vi "Firmware.vi"() -> ()   [LabVIEW 2017]
uses:
  <vilib>/Platform/TimedLoop/XDataNode/timing_clust.ctl
  <vilib>/Platform/TimedLoop/XDataNode/nitl_modes.ctl
  <vilib>/Platform/TimedLoop/XDataNode/wakeup.ctl
  <instrlib>/_niInstr/Instruction Framework/v1/FPGA/Helper Classes/Single Address Space Collection/Single Address Space Collection.lvclass
  C:/Program Files (x86)/National Instruments/LabVIEW 2017/instr.lib/_niInstr/Instruction Framework/v1/FPGA/Interfaces/Address Space Collection/Address Space Collection.lvclass
  <instrlib>/_niInstr/FIFO Register Bus/v1/FPGA/niInstr FIFO Register Bus v1 FPGA.lvclass
  C:/Program Files (x86)/National Instruments/LabVIEW 2017/instr.lib/_niInstr/Instruction Framework/v1/FPGA/Interfaces/Instruction Producer/Instruction Producer.lvclass
  <vilib>/rvi/Emulation/niFpgaGetClockAttributes.vi
  <vilib>/rvi/Emulation/niFpgaSctlEmulationGetInTimedLoop.vi
  <vilib>/rvi/Emulation/niFpgaEmulationReportErrorSimple.vi
  <vilib>/rvi/Emulation/niFpgaProcessEmulError.vi
  <vilib>/rvi/Emulation/niFpgaCriticalErrorInLSC.vi
  <vilib>/rvi/eio/common/nirviEmuTemplateMethod_errors.vi
  <vilib>/eio/EIONode/EIONode.xnode
  <vilib>/Platform/TimedLoop/XDataNode/XDataNode.xnode
  <instrlib>/_niInstr/Instruction Framework/v1/FPGA/Top Level Bus/Register Configuration/Register Configuration.lvclass
  <vilib>/Platform/TimedLoop/XDataNode/XDNodeRunTimeDep.lvlib
  <vilib>/NI/PowerElectronicsControl/ScaleAndLimit/Core/ScaleAndLimit.lvlib
  <vilib>/NI/PowerElectronicsControl/ScaleAndLimit/Core/AddressSpace.lvclass
  <vilib>/NI/PowerElectronicsControl/WaveformAcq/FPGA/WaveformAddressSpace.lvclass
panel:
  in  "ManualTrigger":bool
  out "TriggerTimestamp":i32
  out "FaultBuffer":u64 format="%.0x"
  out "relativeTimestamp":i32
  in  "fifo reg bus ctrl 0":u32
  out "fifo reg bus status 0":u32
  out "fifo reg bus data 0":u64
  out "SimultaneousAILoopRate":u32
  out "LimitsFlag":bool
  out "Simultaneous_AI":sgl[](array[numeric])
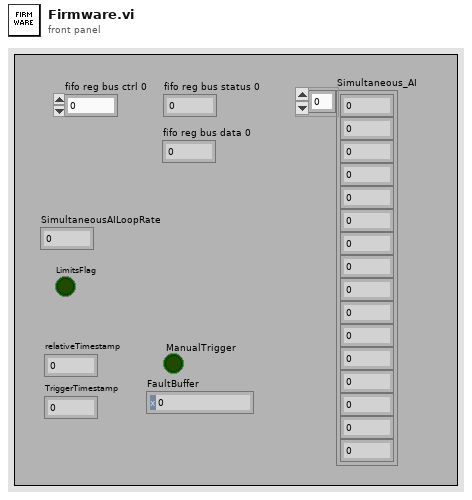
[diagram p1: front panel]
types:
  T1 = typedef "XDNodeRunTimeDep.lvlib/timing_clust.ctl" = cluster{"Expected End [f-1]":u64, "Actual End [f-1]":u64, "Finished Late? [f-1]":bool, "Expected End [i-1]":u64, "Actual End [i-1]":u64, "Finished Late? [i-1]":bool, "Expected Start [i]":u64, "Actual Start [i]":u64, "Expected Start [f]":u64, "Actual Start [f]":u64, "Source Name":string, "Structure Name":string, "Period":i64, "Deadline":i64, "Offset":i64, "Start":i64, "Priority":i32, "Timeout":i32, "Mode":T2, "Wakeup Reason":T3, "Error":errorcluster, "Source Type":string, "Secondary Source Type":string, "Global End Time":u64, "Global Start Time":u64, "Frame Duration":u64, "Iteration Duration":u64, "Assigned CPU":i32, "I/O Scan Engine Mode":u32}
  T2 = typedef "XDNodeRunTimeDep.lvlib/nitl_modes.ctl" = enum32{"No Change", "Process missed periods, maintain original phase", "Discard missed periods, maintain original phase", "Process missed periods, ignore original phase", "Discard missed periods, ignore original phase"}
  T3 = typedef "XDNodeRunTimeDep.lvlib/wakeup.ctl" = enum32{"Normal", "Aborted", "Asynchronous wakeup", "Timing source error", "Timed loop error", "Timeout"}
  T4 = typedef "ScaleAndLimit.lvlib/LimitsRegisters.ctl" = cluster{"HighLimits":refnum<k21>, "LowLimits":refnum<k21>, "ClearLimits":refnum<k21>, "LimitsFlag":refnum<k21>}
  T5 = typedef "ScaleAndLimit.lvlib/ConfigRegisters.ctl" = cluster{"LimitsEnabled":refnum<k21>, "UnscaledHighLimit":refnum<k21>, "UnscaledLowLimit":refnum<k21>, "B":refnum<k21>, "M":refnum<k21>}
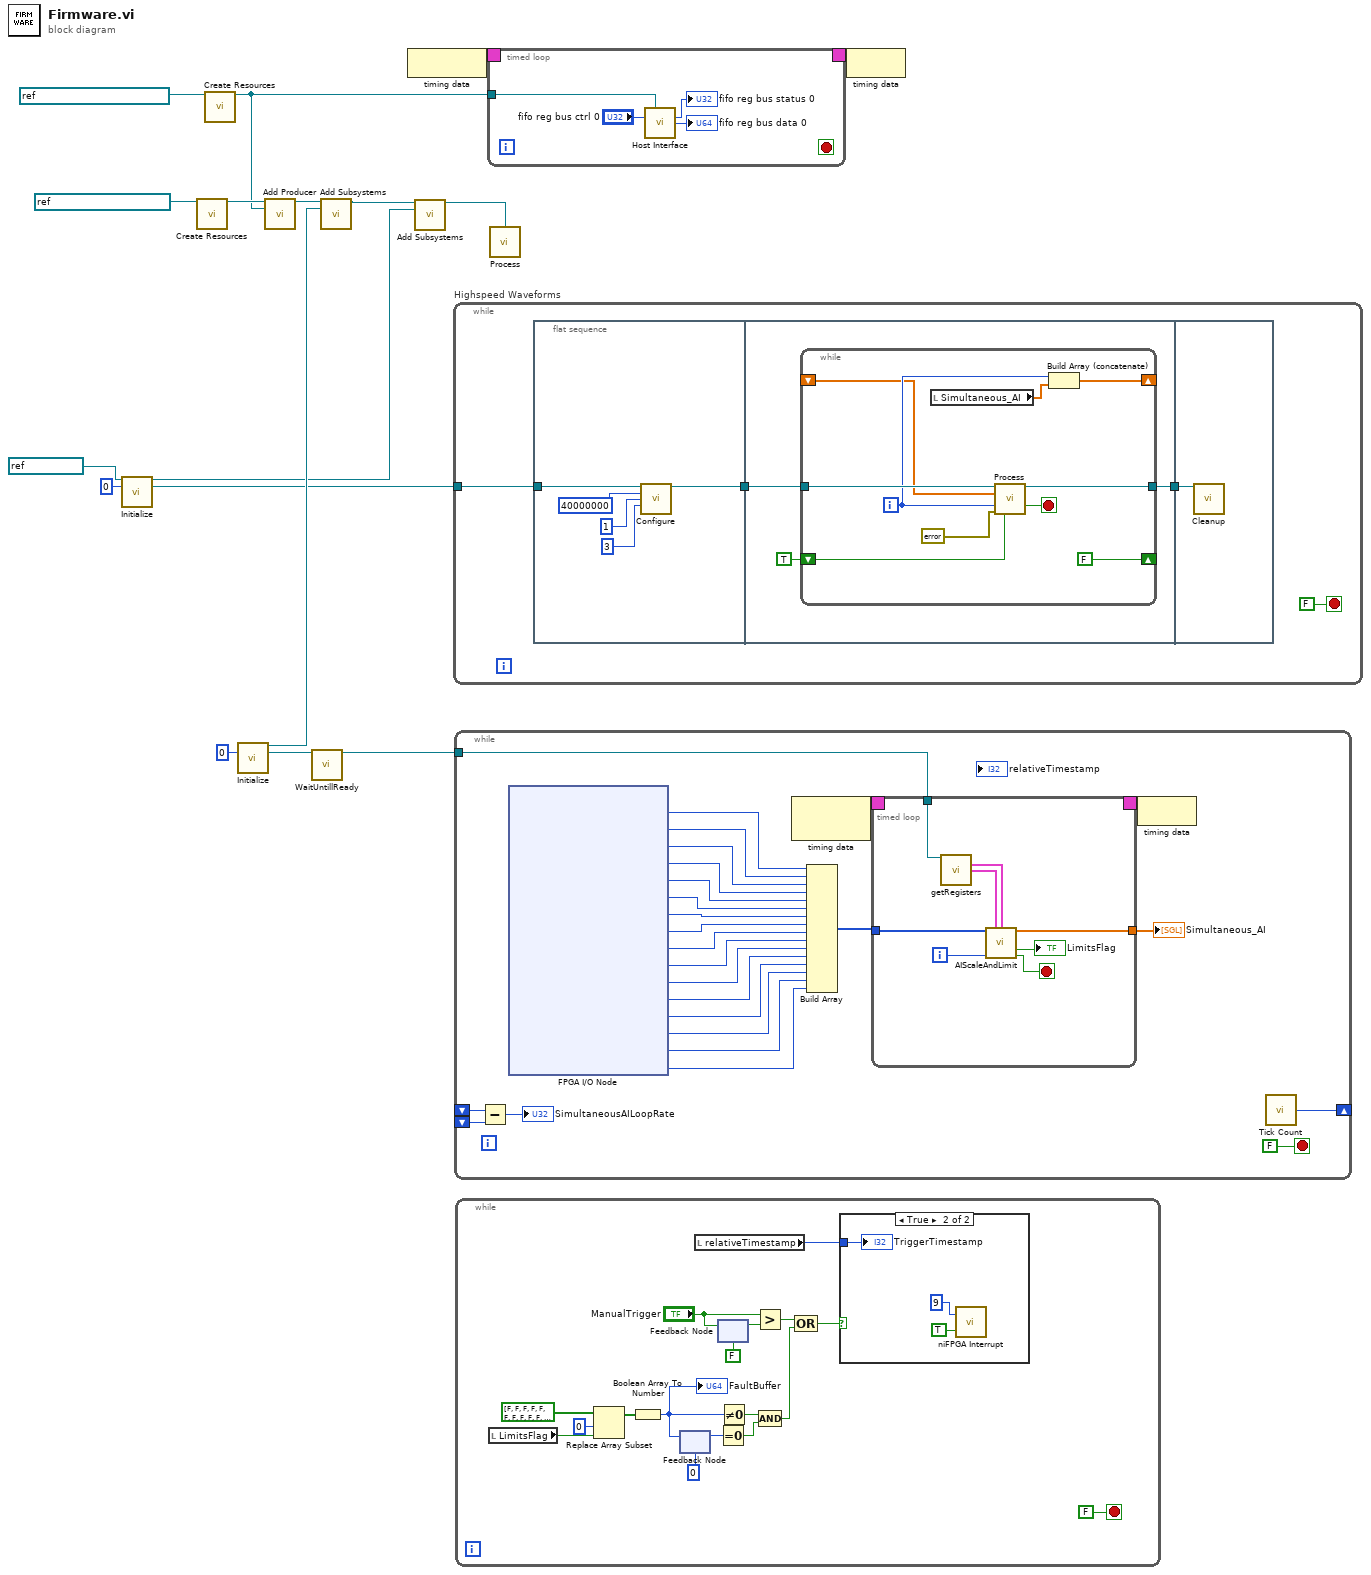
[diagram p0: block diagram]
diagram:
  n1 = call <vilib>:"Initialize.vi"("DMA FIFO"=refnum<k21> "DataSGL0" ("FIFO Out"), "instance"=u8 0) -> ("subsystem"=w3:refnum<class "Single Address Space Collection.lvclass">, "AddressSpace"=w6:refnum<class "WaveformAddressSpace.lvclass">)  [unwired: 12 in]
  n2 = call <instrlib>:"Create Resources.vi"("register clock"=refnum<k21> "40 MHz Onboard Clock") -> ("register configuration"=w15:refnum<class "Register Configuration.lvclass">)  [unwired: 14 in]
  n3 = call <instrlib>:"Create Resources.vi"("instruction fifo"=refnum<k21> "reg.host instruction fifo 0") -> ("fifo register bus"=w7:refnum<class "niInstr FIFO Register Bus v1 FPGA.lvclass">)  [unwired: 14 in]
  n4 = call <vilib>:"Initialize.vi"("instance"=u8 0) -> ("subsystem"=w12:refnum<class "Single Address Space Collection.lvclass">, "AddressSpace"=w10:refnum<class "AddressSpace.lvclass">)  [unwired: 13 in]
  n5 = call <instrlib>:"Add Producer.vi"("register configuration in"=w15, "instruction producer"=w7) -> ("register configuration out"=w13:refnum<class "Register Configuration.lvclass">)  [unwired: 13 in]
  n6 = call <vilib>:"WaitUntillReady.vi"("AddressSpace in"=w10) -> ("AddressSpace out"=w9:refnum<class "AddressSpace.lvclass">)  [unwired: 14 in]
  n7 = call <instrlib>:"Add Subsystems.vi"("register configuration in"=w13, "subsystems"=w12) -> ("register configuration out"=w1:refnum<class "Register Configuration.lvclass">)  [unwired: 13 in]
  n8 = node-c288() -> (w17:T1)
  n9 = call <instrlib>:"Add Subsystems.vi"("register configuration in"=w1, "subsystems"=w3) -> ("register configuration out"=w2:refnum<class "Register Configuration.lvclass">)  [unwired: 13 in]
  n10 = while "Highspeed Waveforms" {
    tunnel: w6 -> [w18]
    stop <- FALSE stop-if-true
    n11 = flat-sequence {
      tunnel: [w22] -> w20
      tunnel: w18 -> [w23]
      tunnel: w20 -> [w29]
      tunnel: [w28] -> w19
      tunnel: w19 -> [w40]
      frame #0 {
        n12 = call <vilib>:"Configure.vi"("WaveformAddressSpace in"=w23, "oclk_freq"=u32 40000000, "oclk_mult"=u32 1, "UnderflowMargin"=u32 3 ("y")) -> ("WaveformAddressSpace out"=w22:refnum<class "WaveformAddressSpace.lvclass">)  [unwired: 11 in]
      }
      frame #1 {
        n13 = while {
          shift-right: [w38] -> _
          shift-left: _ -> [w30]
          shift-right: [FALSE] -> _
          shift-left: TRUE -> [w33]
          tunnel: w29 -> [w35]
          tunnel: [w34] -> w28
          i -> [w32]
          stop <- w36 stop-if-true
          n14 = local read "Simultaneous_AI"() -> (w31:sgl[])
          n15 = call <instrlib>:"Process.vi"("WaveformAddressSpace in"=w35, "Data"=w30, "Iteration"=w32, "error in (no error)"=errorcluster {"status"=FALSE, "code"=0, "source"=""} ("injectError1"), "FirstIteration"=w33) -> ("WaveformAddressSpace out"=w34:refnum<class "WaveformAddressSpace.lvclass">, "stop"=w36:bool)  [unwired: 7 in, 2 out]
          n16 = Build Array (concatenate)(w32, w31) -> (w38:sgl[])
        }
      }
      frame #2 {
        n17 = call <vilib>:"Cleanup.vi"("WaveformAddressSpace in"=w40) -> ()  [unwired: 14 in, 1 out]
      }
    }
  }
  n18 = while {
    shift-right: [w65] -> _
    shift-left: _ -> [w64]
    shift-left: _ -> [w63]
    tunnel: w9 -> [w43]
    stop <- FALSE stop-if-true
    n19 = Subtract(x=w64, y=w63) -> (x-y=→"SimultaneousAILoopRate":u32)
    n20 = xnode "FPGA I/O Node"() -> ("RMC/Simultaneous/AI0"=w61:i16, "RMC/Simultaneous/AI1"=w60:i16, "RMC/Simultaneous/AI2"=w59:i16, "RMC/Simultaneous/AI3"=w58:i16, "RMC/Simultaneous/AI4"=w57:i16, "RMC/Simultaneous/AI5"=w56:i16, "RMC/Simultaneous/AI6"=w55:i16, "RMC/Simultaneous/AI7"=w54:i16, "RMC/Simultaneous/AI8"=w53:i16, "RMC/Simultaneous/AI9"=w52:i16, "RMC/Simultaneous/AI10"=w51:i16, "RMC/Simultaneous/AI11"=w50:i16, "RMC/Simultaneous/AI12"=w49:i16, "RMC/Simultaneous/AI13"=w48:i16, "RMC/Simultaneous/AI14"=w47:i16, "RMC/Simultaneous/AI15"=w41:i16)  [unwired: 16 in, 16 out]
    n21 = node-c288() -> (w46:T1)  [unwired: 1 in]
    n22 = Build Array(w61, w60, w59, w58, w57, w56, w55, w54, w53, w52, w51, w50, w49, w48, w47, w41) -> (w42:i16[])
    n23 = timed-loop {
      timing: w46 -> [_]
      timing-out: [_] -> w45
      tunnel: w42 -> [w74]
      tunnel: [w73] -> w44
      tunnel: w43 -> [w71]
      i -> [w68]
      stop <- w72 stop-if-true
      n24 = call <vilib>:"getRegisters.vi"("AddressSpace in"=w71) -> ("LimitsRegisters"=w69:T4, "ConfigRegisters"=w70:T5)  [unwired: 12 in, 1 out]
      n25 = call <vilib>:"AIScaleAndLimit.vi"("UnscaledAI"=w74, "ConfigRegisters"=w70, "LimitsRegisters"=w69, "index"=w68) -> ("ScaledAI"=w73:sgl[], "Limited"=→"LimitsFlag":bool, "output valid"=w72:bool)  [unwired: 9 in]
    }
    "Simultaneous_AI" <- w44
    n26 = node-c288(w45) -> ()
    n27 = call "Tick Count"() -> ("Tick Count(Ticks)"=w65:u32)
  }
  n28 = while {
    stop <- FALSE stop-if-true
    n29 = local read "LimitsFlag"() -> (w87:bool)
    n30 = Replace Array Subset(array=bool[] [FALSE, FALSE, FALSE, FALSE, FALSE, FALSE, FALSE, FALSE, FALSE, FALSE, FALSE, FALSE, FALSE, FALSE, FALSE, FALSE, FALSE, FALSE, FALSE, FALSE, FALSE, FALSE, FALSE, FALSE, FALSE, FALSE, FALSE, FALSE, FALSE, FALSE, FALSE, FALSE, FALSE, FALSE, FALSE, FALSE, FALSE, FALSE, FALSE, FALSE, FALSE, FALSE, FALSE, FALSE, FALSE, FALSE, FALSE, FALSE, FALSE, FALSE, FALSE, FALSE, FALSE, FALSE, FALSE, FALSE, FALSE, FALSE, FALSE, FALSE, FALSE, FALSE, FALSE, FALSE], new element=w87, index=0) -> (w85:bool[])
    n31 = Boolean Array To Number(Boolean array=w85) -> (number=w83:u64)
    "FaultBuffer" <- w83
    n32 = feedback-in #1(w83) -> ()
    n33 = feedback #1(u64 0) -> (w82:u64)
    n34 = local read "relativeTimestamp"() -> (w89:i32)
    n35 = feedback-in #2("ManualTrigger") -> ()
    n36 = feedback #2(FALSE ("ManualTrigger")) -> (w93:bool)
    n37 = Equal To 0?(x=w82) -> (x = 0?=w80:bool)
    n38 = Not Equal To 0?(x=w83) -> (x != 0?=w81:bool)
    n39 = Greater?(x="ManualTrigger", y=w93) -> (0:w94:bool)
    n40 = Compound Arithmetic op=AND(w81, w80) -> (w79:bool)
    n41 = Compound Arithmetic op=OR(w94, w79) -> (w91:bool)
    n42 = case shown="True" w91 {
      tunnel: w89 -> [_ w96]
      frame False {
      }
      frame True {
        n43 = call <vilib>:"niFPGA Interrupt.vi"("Wait Until Cleared (F)"=TRUE, "IRQ Number (0)"=u8 9) -> ()  [unwired: 1 in]
        "TriggerTimestamp" <- w96
      }
    }
  }
  n44 = timed-loop {
    timing: w17 -> [_]
    timing-out: [_] -> w16
    tunnel: w7 -> [w102]
    stop <- _ stop-if-true
    n45 = call <instrlib>:"Host Interface.vi"("fifo register bus"=w102, "fifo reg bus ctrl 0"="fifo reg bus ctrl 0") -> ("fifo reg bus status 0"=→"fifo reg bus status 0":u32, "fifo reg bus data 0"=→"fifo reg bus data 0":u64)  [unwired: 12 in]
  }
  n46 = call <instrlib>:"Process.vi"("register configuration"=w2) -> ()  [unwired: 15 in]
  n47 = node-c288(w16) -> ()
